vi "Add Service Attribute.vi"(8 "error in (no error)":errorcluster, 10 "RESTful service attribute":T1={"Name"="", "Service Attribute Type"=enum."Path", "Value"=""}, 11 "NI_AB_API_RESTful in":refnum<class "NI_AB_API_RESTful.lvclass">) -> (0 "error out":errorcluster, 3 "NI_AB_API_RESTful out":refnum<class "NI_AB_API_RESTful.lvclass">)   [LabVIEW 2020, in "NI_AB_API_RESTful.lvclass"]
uses:
  <vilib>/AppBuilder/AB_API/RESTful/NI_AB_API_RESTful.lvclass
  <vilib>/AppBuilder/AB_API/RESTful/NI_AB_API_RESTful.lvclass/NI_AB_API_RESTful.ctl
  <vilib>/AppBuilder/AB_API/Build/NI_AB_API_Build.lvclass
  <vilib>/AppBuilder/AB_Classes/RESTful/AB_RESTfulWebService.lvclass
  e:/builds/penguin/labview/branches/2020/dev/dist/vi.lib/AppBuilder/AB_API/Targetfile/NI_AB_API_Targetfile.lvclass
  e:/builds/penguin/labview/branches/2020/dev/dist/vi.lib/AppBuilder/AB_API/Build/NI_AB_API_Build.lvclass
  e:/builds/penguin/labview/branches/2020/dev/dist/vi.lib/AppBuilder/AB_API/RESTful/NI_AB_API_RESTful.lvclass
  e:/builds/penguin/labview/branches/2020/dev/dist/vi.lib/AppBuilder/AB_Classes/WebService/AB_WebService.lvclass
  e:/builds/penguin/labview/branches/2020/dev/dist/vi.lib/AppBuilder/AB_Classes/TargetFile/AB_Targetfile.lvclass
  e:/builds/penguin/labview/branches/2020/dev/dist/vi.lib/AppBuilder/AB_Classes/Build/AB_Build.lvclass
  e:/builds/penguin/labview/branches/2020/dev/dist/vi.lib/AppBuilder/AB_Classes/RESTful/AB_RESTfulWebService.lvclass
  <vilib>/AppBuilder/AB_Classes/RESTful/AB_RESTful_ServiceAttributeType.ctl
  <vilib>/AppBuilder/AB_Classes/RESTful/AB_RESTful_ServiceAttribute.ctl
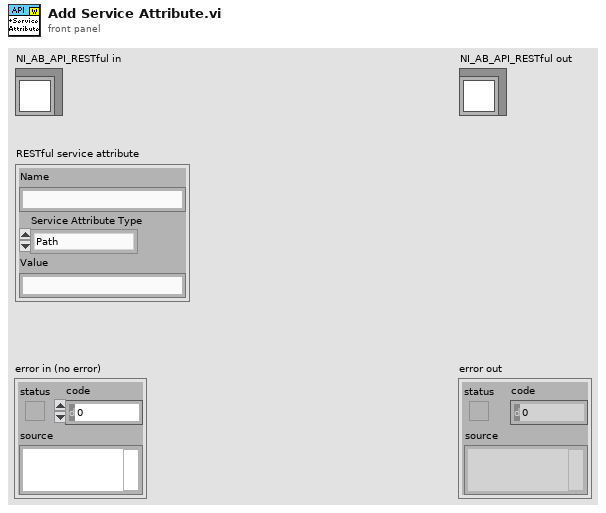
[diagram p1: front panel]
types:
  T1 = typedef "AB_RESTful_ServiceAttribute.ctl" = cluster{"Name":string, "Service Attribute Type":T2, "Value":string}
  T2 = typedef "AB_RESTful_ServiceAttributeType.ctl" = enum32{"String", "Path"}
  T3 = typedef "AB_RESTfulWebService.ctl" = cluster{"routing templates":T4[], "defaultStaticDoc":string, "eng_attributes":T1[], "Privilege Mapping":cluster{"Privilege":string, "Description":string, "Role":string}[]}
  T4 = typedef "AB_RESTful_RoutingTemplate.ctl" = cluster{"Template":string, "Routing Type":T5, "HTTP Method Type":T6, "VIName":string, "Default String":string, "Require API key":bool, "Auth permissions":string[], "eng_Static Alias":string, "Required Privilege":string}
  T5 = typedef "AB_RESTful_RoutingType.ctl" = enum32{"Method", "Static"}
  T6 = typedef "AB_RESTful_HTTPMethodType.ctl" = enum32{"GET", "POST", "PUT", "DELETE"}
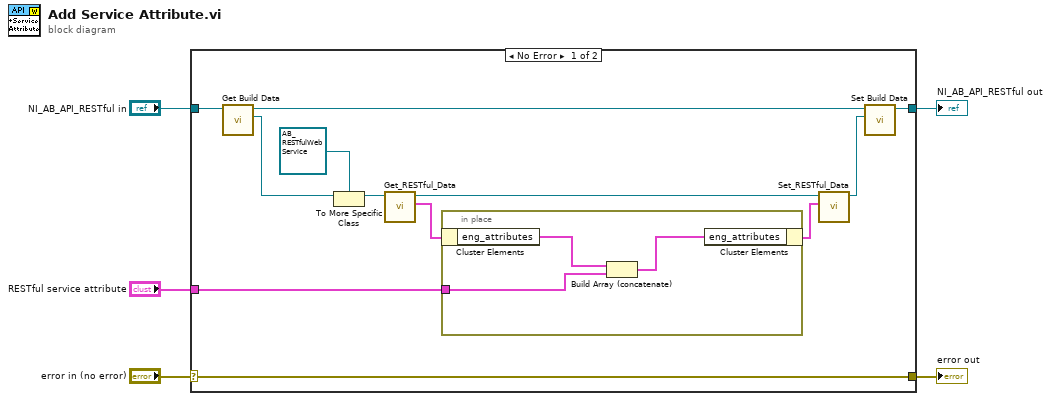
[diagram p0: block diagram]
diagram:
  n1 = case shown="No Error" "error in (no error)" {
    selector: "error in (no error)" -> [w17 w22]
    tunnel: [w17 w22] -> w4
    tunnel: [w14 w21] -> w2
    tunnel: "NI_AB_API_RESTful in" -> [w16 w21]
    tunnel: "RESTful service attribute" -> [w6 _]
    frame No Error {
      n2 = call <vilib>:"Get Build Data.vi"("NI_AB_API_Build in"=w16) -> ("AB_Build.lvclass"=w12:refnum<class "AB_Build.lvclass">, "NI_AB_API_Build out"=w15:refnum<class "NI_AB_API_RESTful.lvclass">)  [unwired: 8 in, 1 out]
      n3 = To More Specific Class(target class=refnum<class "AB_RESTfulWebService.lvclass"> refnum ("AB_RESTfulWebService.lvclass"), reference=w12) -> (specific class reference=w11:refnum<class "AB_RESTfulWebService.lvclass">)  [unwired: 1 in, 1 out]
      n4 = call <vilib>:"Get_RESTful_Data.vi"("Class in"=w11) -> ("data"=w8:T3, "Class out"=w10:refnum<class "AB_RESTfulWebService.lvclass">)  [unwired: 8 in, 1 out]
      n5 = in-place {
        in-place-border: w6 -> [w19]
        n6 = in-place-cluster #1(w8) -> ("eng_attributes"=w20:T1[])
        n7 = Build Array (concatenate)(w20, w19) -> (w18:T1[])
        n8 = in-place-cluster #1("eng_attributes"=w18) -> (w7:T3)
      }
      n9 = call <vilib>:"Set_RESTful_Data.vi"("data"=w7, "Class in"=w10) -> ("Class out"=w9:refnum<class "AB_RESTfulWebService.lvclass">)  [unwired: 8 in, 1 out]
      n10 = call <vilib>:"Set Build Data.vi"("AB_Build.lvclass"=w9, "NI_AB_API_Build in"=w15) -> ("NI_AB_API_Build out"=w14:refnum<class "NI_AB_API_RESTful.lvclass">)  [unwired: 8 in, 1 out]
    }
    frame Error {
    }
  }
  "error out" <- w4
  "NI_AB_API_RESTful out" <- w2
